vi "Convert C to F.vi"(1 "섭씨 온도":dbl) -> (0 "화씨 온도":dbl)   [LabVIEW 2015]
doc: "이 VI는 섭씨 값을 화씨 값으로 변환합니다."
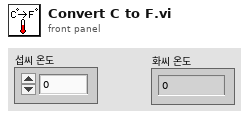
[diagram p1: front panel]
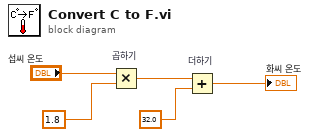
[diagram p0: block diagram]
diagram:
  n1 = Multiply "곱하기"(x="섭씨 온도", y=1.8) -> (x*y=w3:dbl)
  n2 = Add "더하기"(x=w3, y=32.0) -> (x+y=→"화씨 온도":dbl)
